vi "Configure Scan.vi"(6 "Delay Seconds (0 s)":dbl, 7 "Scan Count (1)":u32=1, 8 "error in (no error)":errorcluster, 9 "Channel List(\"\")":string, 10 "Reading Buffer (\"\")":string, 11 "VISA resource name":refnum<visa-resource-name>) -> (0 "error out":errorcluster, 3 "VISA resource name out":refnum<visa-resource-name>)   [LabVIEW 2016, in "Keithley DMM6500 DAQ6500 Series.lvlib"]
doc: "Deletes the existing scan list and creates a new list of channels to scan."
uses:
  Keithley DMM6500 DAQ6500 Series.lvlib
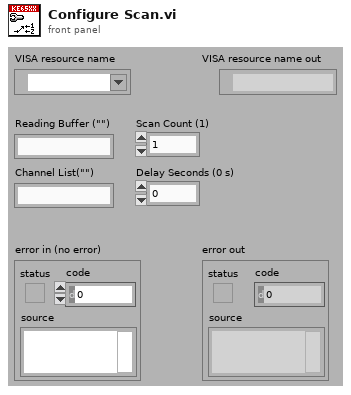
[diagram p1: front panel]
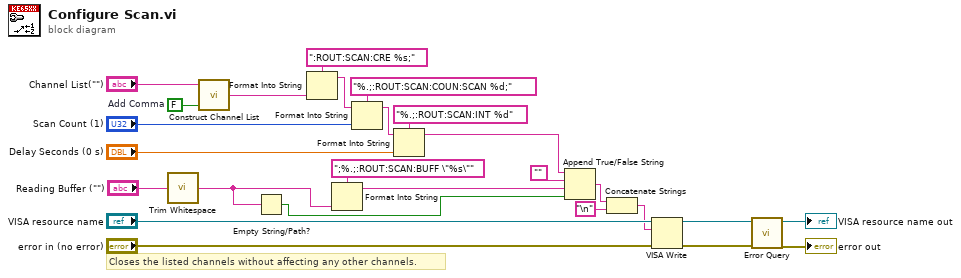
[diagram p0: block diagram]
diagram:
  w17 = FALSE  # Add Comma
  # "Closes the listed channels without affecting any other channels."
  n1 = call <vilib>:"Trim Whitespace.vi"("string"="Reading Buffer (\"\")") -> ("trimmed string"=w1:string)  [unwired: 1 in]
  n2 = call "Construct Channel List.vi"("Add Comma (True)"=w17, "Channel List"="Channel List(\"\")") -> ("Channel List String"=w19:string)  [unwired: 1 in]
  n3 = Empty String/Path?(string/path=w1) -> (empty?=w2:bool)
  n4 = Format Into String(format string=":ROUT:SCAN:CRE %s;", w19) -> (resulting string=w14:string)  [unwired: 2 in, 1 out]
  n5 = Format Into String(format string=";%.;:ROUT:SCAN:BUFF \"%s\"", w1) -> (resulting string=w4:string)  [unwired: 2 in, 1 out]
  n6 = Format Into String(format string="%.;:ROUT:SCAN:COUN:SCAN %d;", initial string=w14, "Scan Count (1)") -> (resulting string=w9:string)  [unwired: 1 in, 1 out]
  n7 = Format Into String(format string="%.;:ROUT:SCAN:INT %d", initial string=w9, "Delay Seconds (0 s)") -> (resulting string=w7:string)  [unwired: 1 in, 1 out]
  n8 = Append True/False String(1:w2, 2:w4, 3:"", 4:w7) -> (0:w6:string)
  n9 = Concatenate Strings(w6, "\n") -> (w16:string)
  n10 = VISA Write(VISA resource name="VISA resource name", write buffer=w16, error in (no error)="error in (no error)") -> (VISA resource name out=w23:refnum<visa-resource-name>, error out=w22:errorcluster)  [unwired: 1 out]
  n11 = call "Error Query.vi"("error in (no error)"=w22, "VISA resource name"=w23) -> ("error out"=→"error out":errorcluster, "VISA resource name out"=→"VISA resource name out":refnum<visa-resource-name>)  [unwired: 6 in, 2 out]
